vi "E_array_index_extractor.vi"(1 "Elements Array":refnum<k21>[](array[refnum]), 2 "True False Array":bool[](array[boolean])) -> (0 "New Elements Array":refnum<k21>[](array[refnum]))   [LabVIEW 2013]
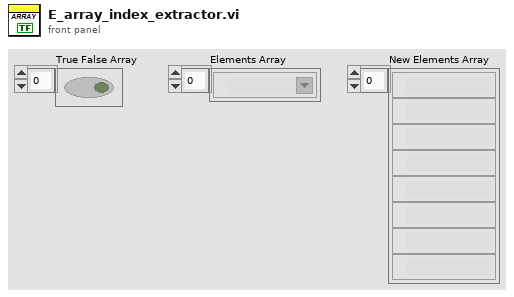
[diagram p1: front panel]
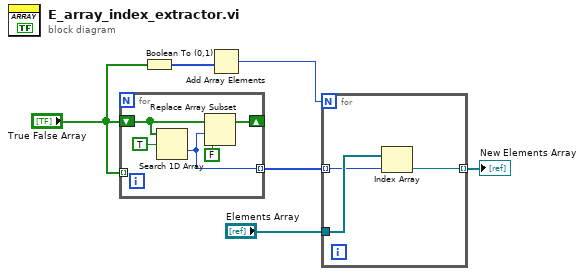
[diagram p0: block diagram]
diagram:
  n1 = for {
    shift-right: [w10] -> _
    shift-left: "True False Array" -> [w9]
    tunnel: [w8] -> w6 mode=indexing
    tunnel: "True False Array" -> [_] mode=indexing
    n2 = Search 1D Array(1D array=w9, element=TRUE) -> (index of element=w8:i32)  [unwired: 1 in]
    n3 = Replace Array Subset(array=w9, new element=FALSE ("new element/subarray"), index=w8) -> (w10:bool[])
  }
  n4 = Boolean To (0,1)(Boolean="True False Array") -> (0, 1=w4:i16[])
  n5 = Add Array Elements(numeric array=w4) -> (sum=w3:i16)
  n6 = for {
    N: w3 -> [_]
    tunnel: w6 -> [w13] mode=indexing
    tunnel: "Elements Array" -> [w14]
    tunnel: [w12] -> w5 mode=indexing
    n7 = Index Array(array=w14, index=w13) -> (element=w12:refnum<k21>)
  }
  "New Elements Array" <- w5
